vi "Set Configuration.vi"(8 "error in (no error)":errorcluster, 10 "Content":refnum<class "Content.lvclass">, 11 "LED Matrix in":refnum<class "LED Matrix.lvclass">) -> (0 "error out":errorcluster, 3 "LED Matrix out":refnum<class "LED Matrix.lvclass">)   [LabVIEW 2026, in "LED Matrix.lvlib" / "LED Matrix.lvclass"]
uses:
  LED Matrix.lvclass
  LED Matrix.lvclass/LED Matrix.ctl
  Content/Content.lvclass
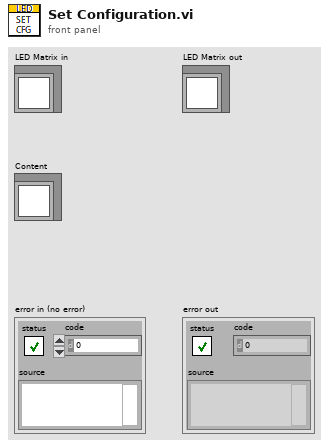
[diagram p1: front panel]
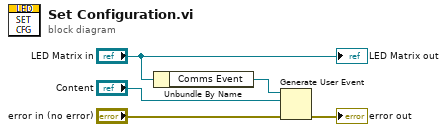
[diagram p0: block diagram]
diagram:
  n1 = Unbundle By Name("LED Matrix in") -> ("Comms Event"=w2:refnum<user-event>)
  n2 = Generate User Event(user event=w2, event data cluster="Content", error in="error in (no error)") -> (error out=→"error out":errorcluster)  [unwired: 1 in, 1 out]
  "LED Matrix out" <- "LED Matrix in"
